vi "Write Best Fit_.vi"(8 "Error In":errorcluster, 10 "Best Fit?":bool, 11 "Test in":refnum<class "Test.lvclass">) -> (0 "Error Out":errorcluster, 3 "Test out":refnum<class "Test.lvclass">)   [LabVIEW 2020, in "Test.lvclass"]
uses:
  Test.lvclass
  Test.lvclass/Test.ctl
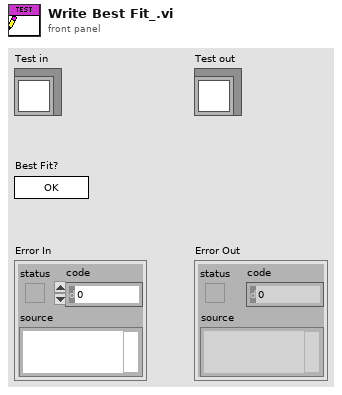
[diagram p1: front panel]
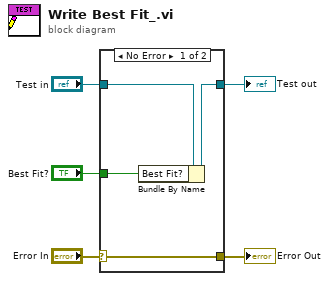
[diagram p0: block diagram]
diagram:
  n1 = case shown="No Error" "Error In" {
    selector: "Error In" -> [w9 w10]
    tunnel: [w9 w10] -> w4
    tunnel: [w7 w11] -> w2
    tunnel: "Test in" -> [w8 w11]
    tunnel: "Best Fit?" -> [w6 _]
    frame No Error {
      n2 = Bundle By Name(cluster=w8, "Best Fit?"=w6) -> (w7:refnum<class "Test.lvclass">)
    }
    frame Error {
    }
  }
  "Error Out" <- w4
  "Test out" <- w2
